vi "client.vi"() -> ()   [LabVIEW 2019]
panel:
  in  "address":string
  in  "values to send":string[](array[string])
  out "echoed values":string[](array[string])
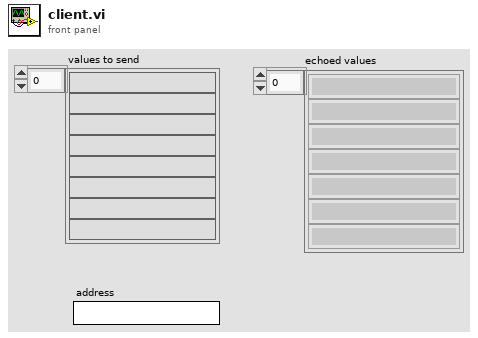
[diagram p1: front panel]
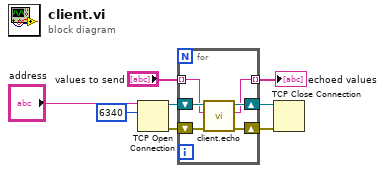
[diagram p0: block diagram]
diagram:
  n1 = TCP Open Connection(address="address", remote port or service name=u16 6340) -> (connection ID=w7:refnum<k5>, error out=w6:errorcluster)  [unwired: 3 in]
  n2 = for {
    tunnel: "values to send" -> [w12] mode=indexing
    tunnel: [w10] -> w3 mode=indexing
    shift-right: [w11] -> w4
    shift-left: w7 -> [w14]
    shift-right: [w9] -> w2
    shift-left: w6 -> [w13]
    n3 = call "client.echo.vi"("error in (no error)"=w13, "value in"=w12, "TCP Network Connection in"=w14) -> ("error out"=w9:errorcluster, "value out"=w10:string, "TCP Network Connection out"=w11:refnum<k5>)  [unwired: 6 in]
  }
  "echoed values" <- w3
  n4 = TCP Close Connection(connection ID=w4, error in (no error)=w2) -> ()  [unwired: 1 in, 2 out]
